vi "SMO.Instrument.TestLauncher.vi"() -> ()   [LabVIEW 2019, in "SMO.Instrument.lvclass"]
doc: "JKI State Machine Objects (SMO) 1.0.0.5\nJKI - JKI\nCopyright (c) 2016, JKI"
uses:
  SMO.Instrument.lvclass
  Typedefs/Data.ctl
  C:/Users/Patrick/Documents/GitHub/Test (LV2019)/lv-venv/lv.lib/vi.lib/JKI/JKI SMO/SMO/SMO.lvclass
  vi.lib/JKI/JKI SMO/SMO/Typedefs/SMOState --Enum.ctl
  vi.lib/JKI/JKI SMO/SMO/SMO.lvclass
panel:
  out "New Value":T1
  in  "Send":bool
  in  "Data":string
  out "error out":errorcluster
  in  "Stop":bool
  # "Intrument Test Launcher"
  # "For instructions on how to use the JKI State Machine Objects, examples and video tutorials, visit:\nhttp://jki.net/state-machine-objects/\n\nJKI State Machine Objects™\nhttp://jki.net/state-machine-objects/\nCopyright (C) 2005-2015, JKI <info@jki.net>\nALL RIGHTS RESERVED"
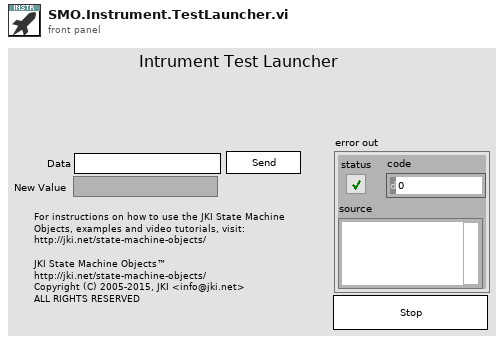
[diagram p1: front panel]
types:
  T1 = typedef "SMO.Instrument.lvclass/Data.ctl" = string
  T2 = typedef "SMO.Instrument.lvclass/PublicEvents--Cluster.ctl" = cluster{"Data Changed":refnum<user-event>}
  T3 = typedef "SMO.lvclass/Public Events.ctl" = cluster{"Error":refnum<user-event>, "State":refnum<user-event>, "Reserve State":refnum<user-event>}
  T4 = typedef "SMO.lvclass/SMOState --Enum.ctl" = enum16{"unknown", "Created", "Started", "Stopped"}
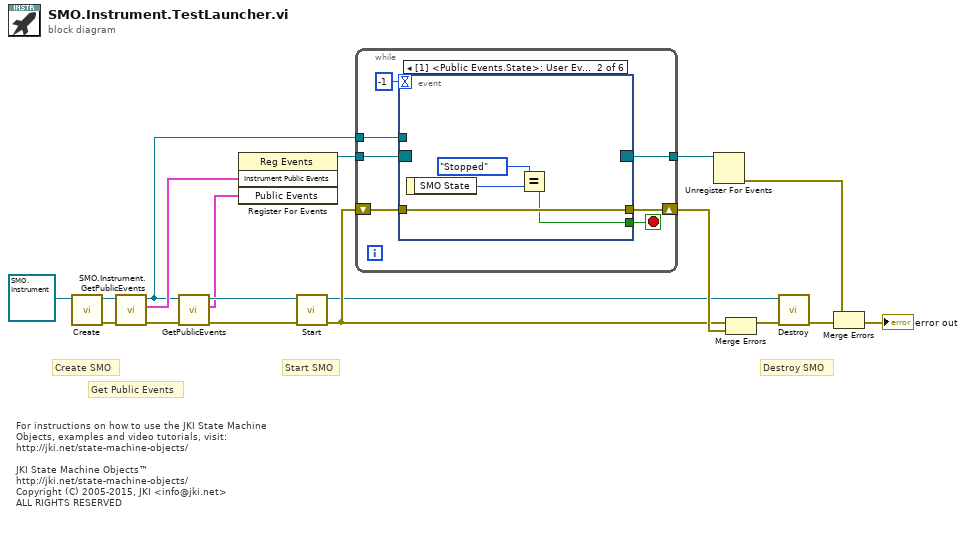
[diagram p0: block diagram]
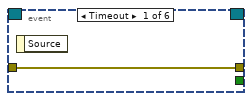
[diagram p2: hidden frame]
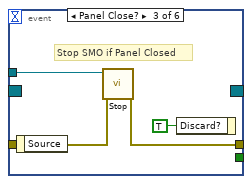
[diagram p3: hidden frame]
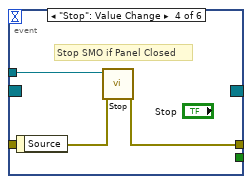
[diagram p4: hidden frame]
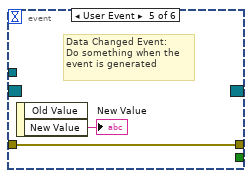
[diagram p5: hidden frame]
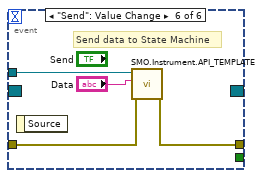
[diagram p6: hidden frame]
diagram:
  # "For instructions on how to use the JKI State Machine Objects, examples and video tutorials, visit:\nhttp://jki.net/state-machine-objects/\n\nJKI State Machine Objects™\nhttp://jki.net/state-machine-objects/\nCopyright (C) 2005-2015, JKI <info@jki.net>\nALL RIGHTS RESERVED"
  # "Get Public Events"
  # "Start SMO"
  # "Destroy SMO"
  # "Create SMO"
  n1 = call "Create.vi"("SMO"=refnum<class "SMO.Instrument.lvclass"> refnum ("SMO.Template.lvclass")) -> ("error out"=w8:errorcluster, "SMO out"=w9:refnum<class "SMO.Instrument.lvclass">)  [unwired: 8 in, 1 out]
  n2 = call "SMO.Instrument.GetPublicEvents.vi"("error in (no error)"=w8, "SMO.Instrument"=w9) -> ("error out"=w3:errorcluster, "Instrument Public Events"=w7:T2, "SMO.Instrument out"=w5:refnum<class "SMO.Instrument.lvclass">)  [unwired: 7 in]
  n3 = call "GetPublicEvents.vi"("error in (no error)"=w3, "SMO"=w5) -> ("error out"=w2:errorcluster, "Public Events"=w1:T3, "SMO out"=w4:refnum<class "SMO.Instrument.lvclass">)  [unwired: 7 in]
  n4 = register-events(w7, w1) -> (reference out=w6:refnum<event-registration>)  [unwired: 2 in, 1 out]
  n5 = call "Start.vi"("error in (no error)"=w2, "SMO"=w4) -> ("error out"=w12:errorcluster, "SMO out"=w10:refnum<class "SMO.Instrument.lvclass">)  [unwired: 8 in]
  n6 = while {
    shift-right: [w24] -> w17
    shift-left: w12 -> [w23]
    tunnel: w6 -> [w22]
    tunnel: [w21] -> w18
    tunnel: w5 -> [w20]
    stop <- w25 stop-if-true
    n7 = event shown="[1] <Public Events.State>: User Event" {
      selector: w22 -> [_ _ _ _ _ _]
      dyn-events: [_ _ _ _ _ _] -> w21
      timeout: -1 -> [_ _ _ _ _ _]
      tunnel: [_ w27 _ _ _ _] -> w25
      tunnel: w20 -> [_ _ w34 w37 _ w43]
      tunnel: [w26 w30 w33 w36 w39 w40] -> w24
      tunnel: w23 -> [w26 w30 w32 w35 w39 w41]
      event Timeout {
        n8 = event-data() -> ()  [unwired: 1 in, 1 out]
      }
      event User Event {
        n9 = event-data() -> ("SMO State"=w29:T4)  [unwired: 1 in]
        n10 = Equal?(x=SMOState_--Enum."Stopped", y=w29) -> (x = y?=w27:bool)
      }
      event Panel Close? {
        # "Stop SMO if Panel Closed"
        n11 = event-data() -> ()  [unwired: 1 in, 1 out]
        n12 = call "Stop.vi"("error in (no error)"=w32, "SMO"=w34) -> ("error out"=w33:errorcluster)  [unwired: 8 in, 1 out]
        n13 = event-data("Discard?"=TRUE ("OK")) -> ()  [unwired: 1 in, 1 out]
      }
      event "Stop": Value Change {
        # "Stop SMO if Panel Closed"
        n14 = event-data() -> ()  [unwired: 1 in, 1 out]
        n15 = call "Stop.vi"("error in (no error)"=w35, "SMO"=w37) -> ("error out"=w36:errorcluster)  [unwired: 8 in, 1 out]
      }
      event User Event {
        # "Data Changed Event:\nDo something when the\nevent is generated"
        n16 = event-data() -> ("New Value"=→"New Value":T1)  [unwired: 1 in, 1 out]
      }
      event "Send": Value Change {
        # "Send data to State Machine"
        n17 = event-data() -> ()  [unwired: 1 in, 1 out]
        n18 = call "SMO.Instrument.API_TEMPLATE.vi"("error in (no error)"=w41, "Data"="Data", "SMO.Instrument"=w43) -> ("error out"=w40:errorcluster)  [unwired: 7 in, 1 out]
      }
    }
  }
  n19 = Unregister For Events(event registration refnum=w18) -> (error out=w16:errorcluster)  [unwired: 1 in]
  n20 = Merge Errors(w12, w17) -> (w11:errorcluster)
  n21 = call "Destroy.vi"("error in (no error)"=w11, "SMO"=w10) -> ("error out"=w14:errorcluster)  [unwired: 9 in]
  n22 = Merge Errors(w16, w14) -> (→"error out":errorcluster)
